vi "CheckValues.vi"(9 "Numeric":i32, 10 "y":dbl, 11 "Cluster in":cluster{"SensorCluster":T1}) -> (2 "Boolean":bool, 3 "Cluster out":cluster{"SensorCluster":T1})   [LabVIEW 2018]
uses:
  Type_Def/Type_Def ClusterSensor.ctl
  Type_Def/Type_Def ControlState.ctl
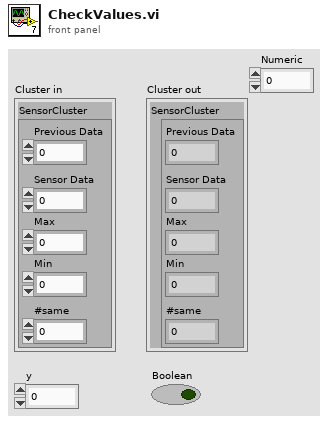
[diagram p1: front panel]
types:
  T1 = typedef "Type_Def ClusterSensor.ctl" = cluster{"Sensor Data":dbl, "Max":dbl, "Min":dbl, "Previous Data":dbl, "#same":dbl}
  T2 = typedef "Type_Def ControlState.ctl" = enum16{"Blank", "Systems Check", "Idle", "Ready", "Pushing", "CrawlingPrecharge", "Braking", "Fault", "Boot Up", "Unpowered", "Crawling", "Shutdown", "Service Push", "Service Wait", "Vent", "Precharge"}
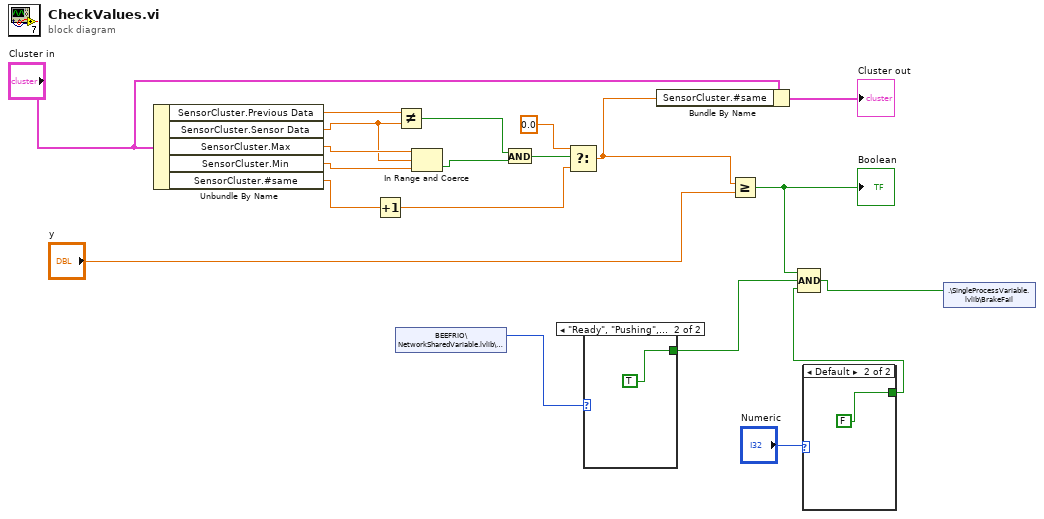
[diagram p0: block diagram]
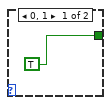
[diagram p2: hidden frame]
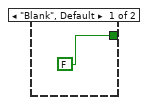
[diagram p3: hidden frame]
diagram:
  n1 = Unbundle By Name("Cluster in") -> ("SensorCluster.Previous Data"=w7:dbl, "SensorCluster.Sensor Data"=w8:dbl, "SensorCluster.Max"=w9:dbl, "SensorCluster.Min"=w10:dbl, "SensorCluster.#same"=w15:dbl)
  n2 = Increment(x=w15) -> (x+1=w16:dbl)
  n3 = Not Equal?(x=w7, y=w8) -> (x != y?=w11:bool)
  n4 = shared-variable "BEEFRIO\\NetworkSharedVariable.lvlib\\CurrentState"() -> (w5:T2)  [unwired: 1 in, 1 out]
  n5 = In Range and Coerce(upper limit=w9, x=w8, lower limit=w10) -> (In Range?=w12:bool)  [unwired: 1 out]
  n6 = And(x=w11, y=w12) -> (x .and. y?=w13:bool)
  n7 = Select(t=0.0, s=w13, f=w16) -> (s? t:f=w18:dbl)
  n8 = case shown="\"Ready\", \"Pushing\", \"Crawling\", \"Service Push\"" w5 {
    tunnel: [FALSE TRUE] -> w4
    frame "Blank", Default {
    }
    frame "Ready", "Pushing", "Crawling", "Service Push" {
    }
  }
  n9 = Bundle By Name(cluster="Cluster in", "SensorCluster.#same"=w18) -> (→"Cluster out":cluster{"SensorCluster":T1})
  n10 = Greater Or Equal?(x=w18, y="y") -> (x >= y?=w6:bool)
  "Boolean" <- w6
  n11 = case shown="Default" "Numeric" {
    tunnel: [TRUE FALSE] -> w2
    frame 0, 1 {
    }
    frame Default {
    }
  }
  n12 = Compound Arithmetic op=AND(w6, w4, w2) -> (w1:bool)
  n13 = shared-variable ".\\SingleProcessVariable.lvlib\\BrakeFail"(w1) -> ()  [unwired: 1 in, 1 out]
